vi "Teleop.vi"(10 "Match Info":T1={"Autonomous Elapsed Seconds"=0.0, "TeleOp Elapsed Seconds"=0.0, "Disabled Elapsed Seconds"=0.0, "Visited Autonomous"=FALSE, "Visited TeleOp"=FALSE, "Visited Disabled"=FALSE, "Autonomous Settings"={"Autonomous Style"=enum."Independent", "VI Refnum"=refnum}}, 11 "Call Context":T2) -> ()   [LabVIEW 2013]
doc: "This VI is called for each TeleOp packet received from the DS where the robot is not disabled. It is often used to read from the joysticks and update I/O or to update setpoints for timed control loops. It should complete and return within 20 milliseconds or it may miss DS packets."
uses:
  <vilib>/Rock Robotics/WPI/DriverStation/WPI_DriverStationDerivedRobotMode.ctl
  <vilib>/Rock Robotics/WPI/DriverStation/WPI_DriverStationMatch Info.ctl
  Robot Global Data.vi
  <vilib>/Rock Robotics/WPI/Solenoid/Deprecated/WPI_SolenoidSetBool.vi
  <vilib>/Rock Robotics/WPI/Joystick/WPI_JoystickGetSetRefNum.vi
  <vilib>/Rock Robotics/WPI/RobotDrive/WPI_RobotDriveGetSetRefNum.vi
panel:
  in  "Stop":bool
  out "Digital Input Value":bool
  out "Numeric 1":dbl(slide) scale=0.0..100.0
  out "Boolean 2":bool
  out "Boolean 1":bool
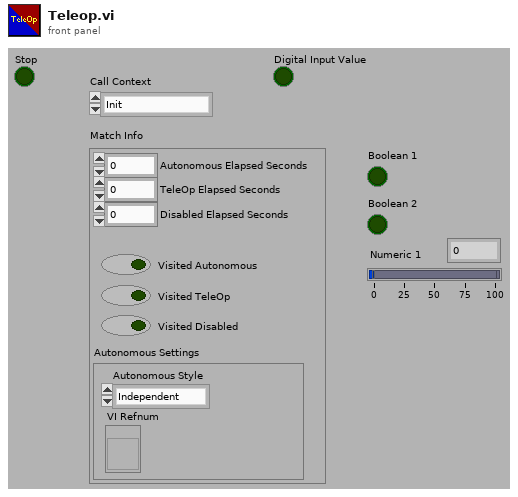
[diagram p1: front panel]
types:
  T1 = typedef "WPI_DriverStationMatch Info.ctl" = cluster{"Autonomous Elapsed Seconds":dbl, "TeleOp Elapsed Seconds":dbl, "Disabled Elapsed Seconds":dbl, "Visited Autonomous":bool, "Visited TeleOp":bool, "Visited Disabled":bool, "Autonomous Settings":cluster{"Autonomous Style":enum16{"Iterative", "Independent"}, "VI Refnum":refnum<vi>}}
  T2 = typedef "WPI_DriverStationDerivedRobotMode.ctl" = enum16{"Init", "Execute", "Stop"}
  T3 = typedef "WPI_JoystickDevRef.ctl" = cluster{"Device":T4}
  T4 = typedef "WPI_JoystickDeviceEnum.ctl" = enum16{"USB 1", "USB 2", "USB 3", "USB 4", "Kinect 1", "Kinect 2"}
  T5 = typedef "WPI_JoystickButtonState.ctl" = cluster{"Button 1":bool, "Button 2":bool, "Button 3":bool, "Button 4":bool, "Button 5":bool, "Button 6":bool, "Button 7":bool, "Button 8":bool, "Button 9":bool, "Button 10":bool, "Button 11":bool, "Button 12":bool}
  T6 = typedef "WPI_SolenoidDevRef.ctl" = cluster{"DevStatus":errorcluster, "Solenoid Module":T7, "Forward Solenoid Channel":T8, "Reverse Solenoid Channel":T8}
  T7 = typedef "FPGA_TypedefSolenoidModule.ctl" = enum16{"Solenoid Module 1", "Solenoid Module 2"}
  T8 = typedef "WPI_SolenoidChannel.ctl" = enum8{"Solenoid 1", "Solenoid 2", "Solenoid 3", "Solenoid 4", "Solenoid 5", "Solenoid 6", "Solenoid 7", "Solenoid 8", "Invalid"}
  T9 = typedef "WPI_MotorControlDeviceRef.ctl" = cluster{"DeviceStatus":errorcluster, "Type":enum16{"PWM", "CAN"}, "PWM":cluster{"Digital Module":T10, "PWM Channel":T11, "DeadBand":T12}, "CAN":cluster{"Device Number":u8, "Control Mode":T13, "Semaphore":T14, "Max Vout":dbl}, "Invert":bool, "TransformRef":T15, "InvTransformRef":T15}
  T10 = typedef "FPGA_TypedefDigitalModule.ctl" = enum16{"Digital Module 1", "Digital Module 2"}
  T11 = typedef "FPGA_DIOPWMChannel.ctl" = enum8{"PWM 1", "PWM 2", "PWM 3", "PWM 4", "PWM 5", "PWM 6", "PWM 7", "PWM 8", "PWM 9", "PWM 10", "Invalid"}
  T12 = typedef "WPI_PWMDeadband.ctl" = cluster{"Name":string, "maxPositivePwm":i32, "minPositivePwm":i32, "centerPwm":i32, "maxNegativePwm":i32, "minNegativePwm":i32, "angularRange":u16}
  T13 = typedef "WPI_CANJaguar_ControlMode.ctl" = enum8{"Percent VBus", "Current", "Speed", "Position", "Voltage"}
  T14 = typedef "Semaphore RefNum" = refnum<k1>
  T15 = typedef "WPI_PWMTransform_ConPane.ctl" = refnum<vi>
  T16 = typedef "WPI_RobotDriveDevRef.ctl" = cluster{"DevStatus":errorcluster, "Motors[]":T9[], "Square Inputs":bool, "Max Output":dbl, "Isochronous":bool}
  T17 = cluster{"axis 1 (x)":dbl, "axis 2 (y)":dbl, "axis 3 (throttle)":dbl, "axis 4":dbl, "axis 5":dbl, "axis 6":dbl}
  T18 = typedef "WPI_DigitalInputDevRef.ctl" = cluster{"DevStatus":errorcluster, "DIO Channel":T19, "Digital Module":T10}
  T19 = typedef "FPGA_DIOChannel.ctl" = enum8{"DIO 1", "DIO 2", "DIO 3", "DIO 4", "DIO 5", "DIO 6", "DIO 7", "DIO 8", "DIO 9", "DIO 10", "DIO 11", "DIO 12", "DIO 13", "DIO 14", "Invalid"}
  T20 = typedef "WPI_RelayDevRef.ctl" = cluster{"DevStatus":errorcluster, "Relay Channel":T21, "Digital Module":T10, "Relay Direction":T22}
  T21 = typedef "FPGA_DIORelayChannel.ctl" = enum8{"Relay 1", "Relay 2", "Relay 3", "Relay 4", "Relay 5", "Relay 6", "Relay 7", "Relay 8", "Invalid"}
  T22 = typedef "WPI_RelayDirection.ctl" = enum16{"Both directions", "Forward only", "Reverse only"}
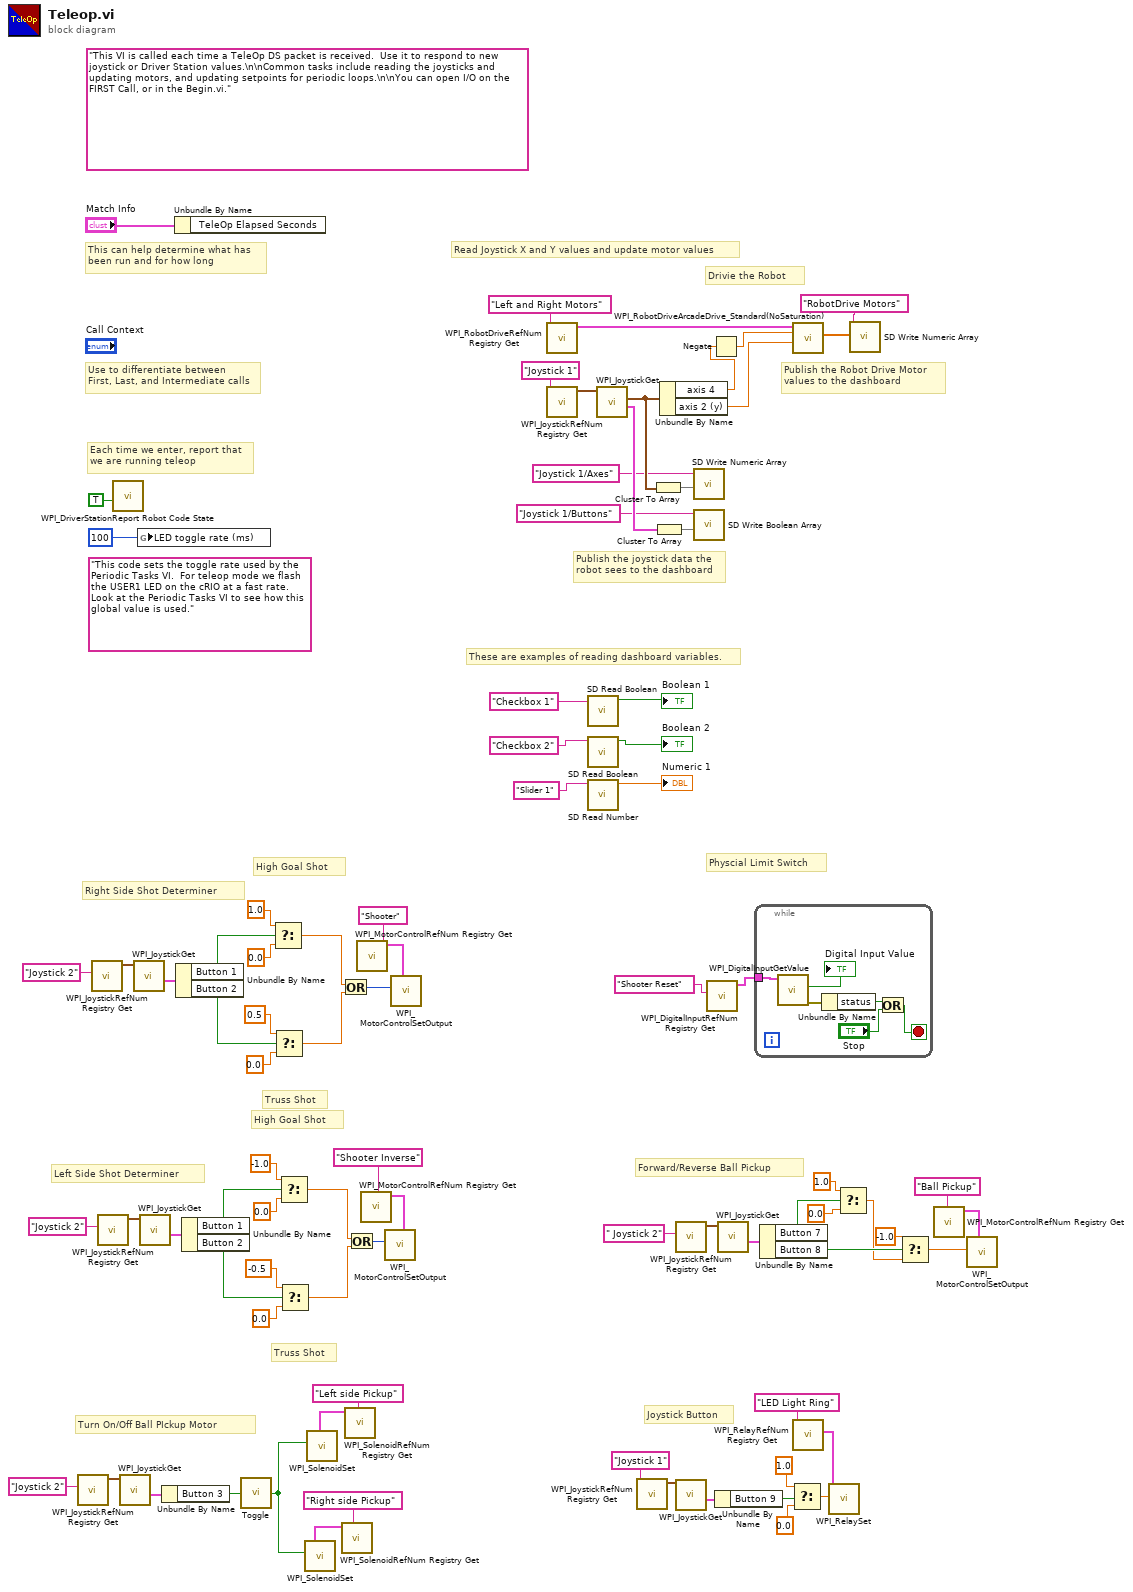
[diagram p0: block diagram]
diagram:
  (unwired) "This code sets the toggle rate used by the Periodic Tasks VI.  For teleop mode we flash the USER1 LED on the cRIO at a fast rate.  Look at the Periodic Tasks VI to see how this global value is used."
  (unwired) "This VI is called each time a TeleOp DS packet is received.  Use it to respond to new joystick or Driver Station values.\n\nCommon tasks include reading the joysticks and updating motors, and updating setpoints for periodic loops.\n\nYou can open I/O on the FIRST Call, or in the Begin.vi."
  # "Turn On/Off Ball PIckup Motor"
  # "Forward/Reverse Ball Pickup"
  # "Truss Shot"
  # "High Goal Shot"
  # "Left Side Shot Determiner"
  # "Truss Shot"
  # "High Goal Shot"
  # "Right Side Shot Determiner"
  # "Physcial Limit Switch"
  # "Joystick Button"
  # "Drivie the Robot"
  # "These are examples of reading dashboard variables."
  # "Publish the Robot Drive Motor\nvalues to the dashboard"
  # "Publish the joystick data the\nrobot sees to the dashboard"
  # "Each time we enter, report that\nwe are running teleop"
  # "Use to differentiate between\nFirst, Last, and Intermediate calls"
  # "This can help determine what has\nbeen run and for how long"
  # "Read Joystick X and Y values and update motor values"
  n1 = call <vilib>:"WPI_JoystickRefNum Registry Get.vi"("refnum name"="Joystick 2") -> ("JoystickDevRef"=w28:T3)  [unwired: 9 in, 1 out]
  n2 = call <vilib>:"WPI_JoystickRefNum Registry Get.vi"("refnum name"="Joystick 2") -> ("JoystickDevRef"=w51:T3)  [unwired: 9 in, 1 out]
  n3 = call <vilib>:"WPI_JoystickRefNum Registry Get.vi"("refnum name"="Joystick 2") -> ("JoystickDevRef"=w5:T3)  [unwired: 9 in, 1 out]
  n4 = call <vilib>:"WPI_DriverStationReport Robot Code State.vi"("TeleOp"=TRUE ("Autonomous")) -> ()  [unwired: 10 in, 1 out]
  n5 = call <vilib>:"WPI_JoystickGet.vi"("JoystickDevRef"=w28) -> ("Buttons"=w27:T5)  [unwired: 4 in, 2 out]
  n6 = call <vilib>:"WPI_JoystickGet.vi"("JoystickDevRef"=w51) -> ("Buttons"=w50:T5)  [unwired: 4 in, 2 out]
  n7 = global write "Robot Global Data.vi" "LED toggle rate (ms)"(u32 100 ("LED ms toggle rate")) -> ()
  n8 = call <vilib>:"WPI_JoystickGet.vi"("JoystickDevRef"=w5) -> ("Buttons"=w6:T5)  [unwired: 4 in, 2 out]
  n9 = Unbundle By Name(w27) -> ("Button 3"=w22:bool)
  n10 = Unbundle By Name("Match Info") -> ()  [unwired: 1 out]
  n11 = Unbundle By Name(w50) -> ("Button 1"=w45:bool, "Button 2"=w44:bool)
  n12 = Unbundle By Name(w6) -> ("Button 1"=w10:bool, "Button 2"=w11:bool)
  n13 = call "Toggle.vi"("Input"=w22) -> ("Toggled Output"=w21:bool)
  n14 = Select(t=1.0, s=w45, f=0.0) -> (s? t:f=w16:dbl)
  n15 = Select(t=0.5, s=w44, f=0.0) -> (s? t:f=w15:dbl)
  n16 = Select(t=-1.0, s=w10, f=0.0) -> (s? t:f=w12:dbl)
  n17 = Select(t=-0.5, s=w11, f=0.0) -> (s? t:f=w13:dbl)
  n18 = Or(x=w16, y=w15) -> (x .or. y?=w14:i32)
  n19 = call <vilib>:"WPI_SolenoidRefNum Registry Get.vi"("refnum name"="Right side Pickup") -> ("SolenoidDevRef"=w25:T6)  [unwired: 9 in, 1 out]
  n20 = call-poly <vilib>:"WPI_SolenoidSet.vi"("Value"=w21, "SolenoidDevRef"=w25) -> ()  [unwired: 8 in, 2 out]
  n21 = call <vilib>:"WPI_SolenoidRefNum Registry Get.vi"("refnum name"="Left side Pickup") -> ("SolenoidDevRef"=w26:T6)  [unwired: 9 in, 1 out]
  n22 = call-poly <vilib>:"WPI_SolenoidSet.vi"("Value"=w21, "SolenoidDevRef"=w26) -> ()  [unwired: 8 in, 2 out]
  n23 = Or(x=w12, y=w13) -> (x .or. y?=w1:i32)
  n24 = call <vilib>:"WPI_MotorControlRefNum Registry Get.vi"("refnum name"="Shooter") -> ("MotorControlDevRef"=w17:T9)  [unwired: 9 in, 1 out]
  n25 = call <vilib>:"WPI_MotorControlRefNum Registry Get.vi"("refnum name"="Shooter Inverse") -> ("MotorControlDevRef"=w3:T9)  [unwired: 9 in, 1 out]
  n26 = call <vilib>:"WPI_MotorControlSetOutput.vi"("Output"=w1, "MotorControlDevRef"=w3) -> ()  [unwired: 7 in, 3 out]
  n27 = call <vilib>:"WPI_MotorControlSetOutput.vi"("Output"=w14, "MotorControlDevRef"=w17) -> ()  [unwired: 7 in, 3 out]
  n28 = call <vilib>:"WPI_RobotDriveRefNum Registry Get.vi"("refnum name"="Left and Right Motors") -> ("RobotDriveDevRef"=w82:T16)  [unwired: 1 in, 9 out]
  n29 = call <vilib>:"WPI_JoystickRefNum Registry Get.vi"("refnum name"="Joystick 1") -> ("JoystickDevRef"=w79:T3)  [unwired: 1 in, 9 out]
  n30 = call <vilib>:"SD Read Boolean.vi"("Name"="Checkbox 1" ("refnum name")) -> ("Boolean"=→"Boolean 1":bool)  [unwired: 8 in, 2 out]
  n31 = call <vilib>:"SD Read Boolean.vi"("Name"="Checkbox 2" ("refnum name")) -> ("Boolean"=→"Boolean 2":bool)  [unwired: 8 in, 2 out]
  n32 = call <vilib>:"SD Read Number.vi"("Name"="Slider 1" ("refnum name")) -> ("Numeric"=→"Numeric 1":dbl)  [unwired: 8 in, 2 out]
  n33 = call <vilib>:"WPI_JoystickGet.vi"("JoystickDevRef"=w79) -> ("Buttons"=w76:T5, "Axes"=w73:T17)  [unwired: 1 in, 4 out]
  n34 = call <vilib>:"WPI_JoystickRefNum Registry Get.vi"("refnum name"="Joystick 1") -> ("JoystickDevRef"=w58:T3)  [unwired: 9 in, 1 out]
  n35 = Cluster To Array(cluster=w73) -> (array=w72:dbl[])
  n36 = Cluster To Array(cluster=w76) -> (array=w75:bool[])
  n37 = Unbundle By Name(w73) -> ("axis 4"=w24:dbl, "axis 2 (y)"=w81:dbl)
  n38 = call <vilib>:"WPI_JoystickRefNum Registry Get.vi"("refnum name"=" Joystick 2") -> ("JoystickDevRef"=w42:T3)  [unwired: 9 in, 1 out]
  n39 = call <vilib>:"WPI_JoystickGet.vi"("JoystickDevRef"=w58) -> ("Buttons"=w57:T5)  [unwired: 4 in, 2 out]
  n40 = call <vilib>:"SD Write Numeric Array.vi"("Numeric Array"=w72, "Name"="Joystick 1/Axes") -> ()  [unwired: 8 in, 2 out]
  n41 = call <vilib>:"SD Write Boolean Array.vi"("Boolean Array"=w75, "Name"="Joystick 1/Buttons") -> ()  [unwired: 8 in, 2 out]
  n42 = call <vilib>:"WPI_DigitalInputRefNum Registry Get.vi"("refnum name"="Shooter Reset") -> ("DigitalInputDevRef"=w18:T18)  [unwired: 9 in, 1 out]
  n43 = Negate(x=w24) -> (-x=w23:dbl)
  n44 = Unbundle By Name(w57) -> ("Button 9"=w56:bool)
  n45 = call <vilib>:"WPI_JoystickGet.vi"("JoystickDevRef"=w42) -> ("Buttons"=w41:T5)  [unwired: 4 in, 2 out]
  n46 = while {
    tunnel: w18 -> [w86]
    stop <- w85 stop-if-true
    n47 = call <vilib>:"WPI_DigitalInputGetValue.vi"("DigitalInputDevRef"=w86) -> ("error out"=w89:errorcluster, "Value"=→"Digital Input Value":bool)  [unwired: 8 in, 1 out]
    n48 = Unbundle By Name(w89) -> ("status"=w87:bool)
    n49 = Or(x=w87, y="Stop") -> (x .or. y?=w85:bool)
  }
  n50 = Unbundle By Name(w41) -> ("Button 7"=w40:bool, "Button 8"=w39:bool)
  n51 = Select(t=1.0, s=w56, f=0.0) -> (s? t:f=w55:dbl)
  n52 = call <vilib>:"WPI_RobotDriveArcadeDrive_Standard(NoSaturation).vi"("Y axis value"=w81, "X axis value"=w23, "RobotDriveDevRef"=w82) -> ("Motor Values"=w69:dbl[])  [unwired: 1 in, 7 out]
  n53 = call <vilib>:"WPI_RelayRefNum Registry Get.vi"("refnum name"="LED Light Ring") -> ("RelayDevRef"=w62:T20)  [unwired: 9 in, 1 out]
  n54 = call <vilib>:"WPI_RelaySet.vi"("RelayValue"=w55, "RelayDevRef"=w62) -> ()  [unwired: 8 in, 2 out]
  n55 = Select(t=1.0, s=w40, f=0.0) -> (s? t:f=w33:dbl)
  n56 = call <vilib>:"SD Write Numeric Array.vi"("Numeric Array"=w69, "Name"="RobotDrive Motors") -> ()  [unwired: 8 in, 2 out]
  n57 = Select(t=-1.0, s=w39, f=w33) -> (s? t:f=w32:dbl)
  n58 = call <vilib>:"WPI_MotorControlRefNum Registry Get.vi"("refnum name"="Ball Pickup") -> ("MotorControlDevRef"=w34:T9)  [unwired: 9 in, 1 out]
  n59 = call <vilib>:"WPI_MotorControlSetOutput.vi"("Output"=w32, "MotorControlDevRef"=w34) -> ()  [unwired: 7 in, 3 out]
